vi "Write Measured Table.vi"(8 "error in (no error)":errorcluster, 10 "Measured Table":refnum<vi>, 11 "Analog-Output in":refnum<class "Analog-Output.lvclass">) -> (0 "error out":errorcluster, 3 "Analog-Output out":refnum<class "Analog-Output.lvclass">)   [LabVIEW 2019, in "Analog-Output.lvlib" / "Analog-Output.lvclass"]
uses:
  Library/Analog-Output.lvclass
  Library/Analog-Output.lvclass/Analog-Output.ctl
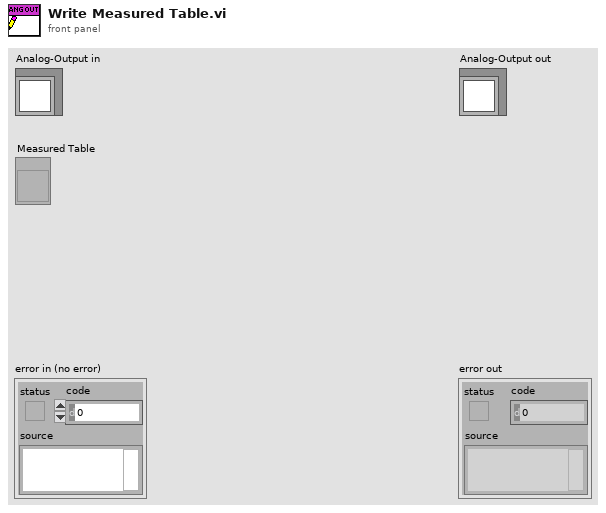
[diagram p1: front panel]
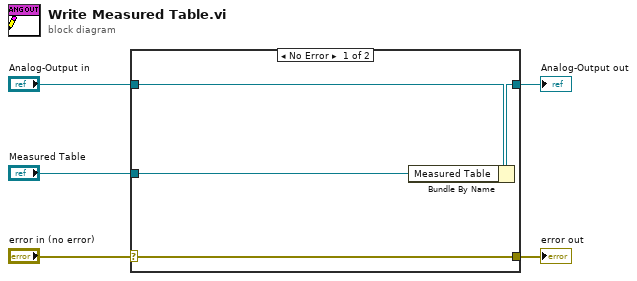
[diagram p0: block diagram]
diagram:
  n1 = case shown="No Error" "error in (no error)" {
    selector: "error in (no error)" -> [w9 w10]
    tunnel: [w9 w10] -> w4
    tunnel: [w7 w11] -> w2
    tunnel: "Analog-Output in" -> [w8 w11]
    tunnel: "Measured Table" -> [w6 _]
    frame No Error {
      n2 = Bundle By Name(cluster=w8, "Measured Table"=w6) -> (w7:refnum<class "Analog-Output.lvclass">)
    }
    frame Error {
    }
  }
  "error out" <- w4
  "Analog-Output out" <- w2
